vi "DecisionMaker.vi"(8 "Goal location":T3 {"North" format="%#_10f"; "East" format="%#_8f"}, 9 "Heading to test":dbl) -> (1 "Heading Goodness":T1)   [LabVIEW 2011]
doc: "VI to make decisions when the boat is headed upwind.\n\nCalculates the vector that goes to the goal from the boat's current location when first called.\nConstantly calculates the two optimal angles with respect to the wind and gives one of them as the optimal angle. On first call, this will be the one that is closer to the robot's current heading. It also calculates the distance from the boat to the original line calculated. If the distance gets larger than the allowed distance, it switches the angle outputted as optimal to the other angle that is good with respect to the wind."
uses:
  2 Typedefs/apparent wind direction.ctl
  2 Globals/2 TuningConstants.vi
  2 Globals/2 Global.vi
panel:
  in  "Irons direct vector":T2 {"Origin"."North" format="%#_10f"; "Origin"."East" format="%#_8f"}
  in  "Already Upwind?":bool
  # "0 < A < 1"
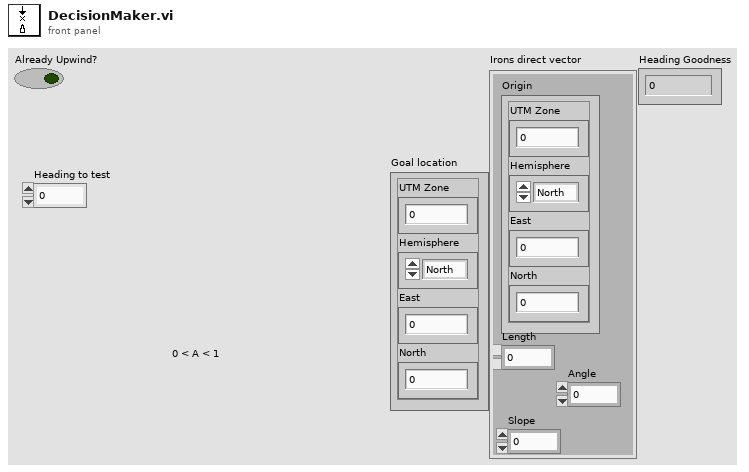
[diagram p1: front panel]
types:
  T1 = typedef "apparent wind direction.ctl" = dbl
  T2 = cluster{"Origin":cluster{"UTM Zone":dbl, "Hemisphere":enum16{"North", "South"}, "East":dbl, "North":dbl}, "Length":dbl, "Angle":dbl, "Slope":dbl}
  T3 = cluster{"UTM Zone":dbl, "Hemisphere":enum16{"North", "South"}, "East":dbl, "North":dbl}
  T4 = typedef "UTM Location.ctl" = cluster{"UTM Zone":dbl, "Hemisphere":enum16{"North", "South"}, "East":dbl, "North":dbl}
  T5 = cluster{"UTM Zone":bool, "Hemisphere":bool, "East":bool, "North":bool}
  T6 = typedef "heading.ctl" = dbl
  T7 = typedef "absolute wind direction.ctl" = dbl
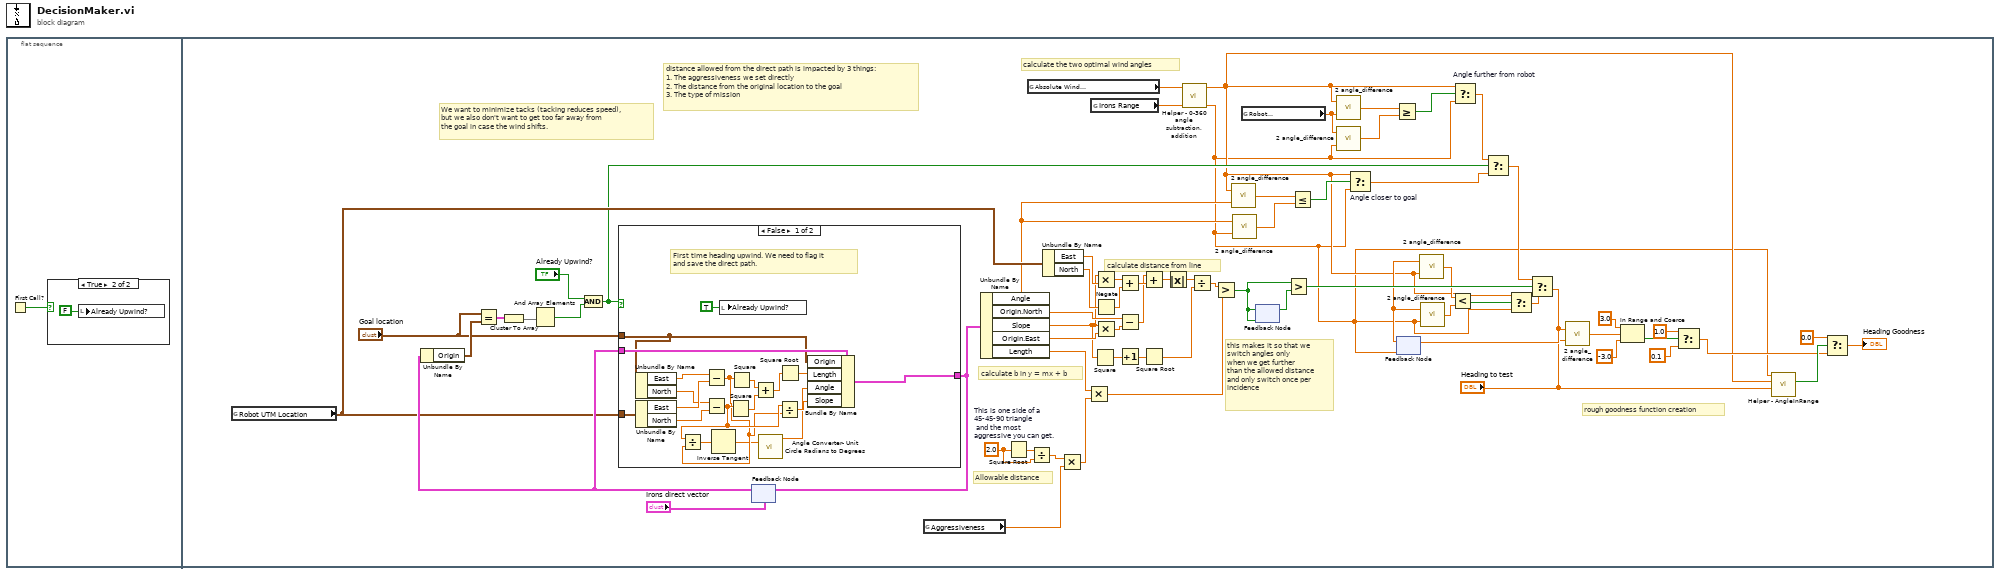
[diagram p0: block diagram]
diagram:
  n1 = flat-sequence {
    frame #0 {
      n2 = First Call?() -> (First Call?: T/F=w1:bool)
      n3 = case shown="True" w1 {
        frame False {
        }
        frame True {
          n4 = local write "Already Upwind?"(FALSE ("Already Upwind?")) -> ()
        }
      }
    }
    frame #1 {
      w47 = 2.0 ("x")
      # "Allowable distance"
      # "rough goodness function creation"
      # "this makes it so that we\nswitch angles only\nwhen we get further\nthan the allowed distance\nand only switch once per\nincidence"
      # "calculate distance from line"
      # "calculate the two optimal wind angles"
      # "calculate b in y = mx + b"
      # "distance allowed from the direct path is impacted by 3 things:\n1. The aggressiveness we set directly\n2. The distance from the original location to the goal\n3. The type of mission"
      # "We want to minimize tacks (tacking reduces speed),\nbut we also don't want to get too far away from\nthe goal in case the wind shifts."
      n5 = global read "2 Global.vi" "Robot UTM Location"() -> (w36:T4)
      n6 = feedback #1("Irons direct vector") -> (w45:T2)
      n7 = Unbundle By Name(w45) -> ("Origin"=w44:T3)
      n8 = Equal?(x="Goal location", y=w44) -> (x = y?=w43:T5)
      n9 = Cluster To Array(cluster=w43) -> (array=w42:bool[])
      n10 = And Array Elements(Boolean array=w42) -> (logical AND=w41:bool)
      n11 = And(x="Already Upwind?", y=w41) -> (x .and. y?=w13:bool)
      n12 = case shown="False" w13 {
        tunnel: w45 -> [w89 w91]
        tunnel: "Goal location" -> [w84 _]
        tunnel: w36 -> [w83 _]
        tunnel: [w77 w91] -> w55
        frame False {
          # "First time heading upwind. We need to flag it\nand save the direct path."
          n13 = Unbundle By Name(w84) -> ("East"=w82:dbl, "North"=w80:dbl)
          n14 = Unbundle By Name(w83) -> ("East"=w81:dbl, "North"=w79:dbl)
          n15 = Subtract(x=w82, y=w81) -> (x-y=w74:dbl)
          n16 = Subtract(x=w80, y=w79) -> (x-y=w75:dbl)
          n17 = Divide(x=w75, y=w74) -> (x/y=w78:dbl)
          n18 = Inverse Tangent(1:w78) -> (0:w73:dbl)
          n19 = local write "Already Upwind?"(TRUE ("Already Upwind?")) -> ()
          n20 = Square(x=w75) -> (x^2=w87:dbl)
          n21 = Square(x=w74) -> (x^2=w88:dbl)
          n22 = Add(x=w88, y=w87) -> (x+y=w85:dbl)
          n23 = call "Angle Converter- Unit Circle Radians to Degrees.vi"("Angle in \nUnit Circle\nRadians"=w73) -> ("Angle in \nHeading \nFormat"=w72:T6)  [unwired: 10 in]
          n24 = Divide(x=w75, y=w74) -> (x/y=w76:dbl)
          n25 = Square Root(x=w85) -> (sqrt(x)=w86:dbl)
          n26 = Bundle By Name(cluster=w89, "Origin"=w84, "Length"=w86, "Angle"=w72, "Slope"=w76) -> (w77:T2)
        }
        frame True {
        }
      }
      n27 = feedback-in #1(w55) -> ()
      n28 = global read "2 TuningConstants.vi" "Aggressiveness"() -> (w26:dbl)
      n29 = Unbundle By Name(w55) -> ("Angle"=w14:dbl, "Origin.North"=w70:dbl, "Slope"=w58:dbl, "Origin.East"=w69:dbl, "Length"=w50:dbl)
      n30 = Square Root(x=w47) -> (sqrt(x)=w48:dbl)
      n31 = global read "2 Global.vi" "Absolute Wind\nDirection (º)"() -> (w30:T7)
      n32 = Divide "This is one side of a 45-45-90 triangle\n and the most aggressive you can get."(x=w48, y=w47) -> (x/y=w29:dbl)
      n33 = Unbundle By Name(w36) -> ("East"=w67:dbl, "North"=w65:dbl)
      n34 = Multiply(x=w29, y=w26) -> (x*y=w28:dbl)
      n35 = Multiply(x=w50, y=w28) -> (x*y=w49:dbl)
      n36 = global read "2 TuningConstants.vi" "Irons Range"() -> (w31:dbl)
      n37 = Square(x=w58) -> (x^2=w57:dbl)
      n38 = Multiply(x=w58, y=w67) -> (x*y=w66:dbl)
      n39 = Negate(x=w65) -> (-x=w64:dbl)
      n40 = Multiply(x=w58, y=w69) -> (x*y=w68:dbl)
      n41 = Add(x=w66, y=w64) -> (x+y=w63:dbl)
      n42 = Subtract(x=w70, y=w68) -> (x-y=w62:dbl)
      n43 = Increment(x=w57) -> (x+1=w56:dbl)
      n44 = Add(x=w62, y=w63) -> (x+y=w61:dbl)
      n45 = Square Root(x=w56) -> (sqrt(x)=w59:dbl)
      n46 = Absolute Value(x=w61) -> (abs(x)=w60:dbl)
      n47 = call "Helper - 0-360 angle subtraction, addition.vi"("y"=w31, "x"=w30) -> ("x + y"=w4:dbl, "x - y"=w5:T1)  [unwired: 8 in]
      n48 = Divide(x=w60, y=w59) -> (x/y=w54:dbl)
      n49 = Greater?(x=w54, y=w49) -> (0:w34:bool)
      n50 = call "2 angle_difference.vi"("Angle 2"=w14, "Angle 1"=w5) -> ("Difference"=w16:dbl)
      n51 = call "2 angle_difference.vi"("Angle 2"=w4, "Angle 1"=w14) -> ("Difference"=w17:dbl)
      n52 = global read "2 Global.vi" "Robot\nHeading"() -> (w23:T6)
      n53 = feedback #2(w34) -> (w33:bool)
      n54 = feedback-in #2(w34) -> ()
      n55 = Greater?(x=w34, y=w33) -> (0:w32:bool)
      n56 = Less Or Equal?(x=w16, y=w17) -> (x <= y?=w15:bool)
      n57 = call "2 angle_difference.vi"("Angle 2"=w23, "Angle 1"=w5) -> ("Difference"=w24:dbl)
      n58 = call "2 angle_difference.vi"("Angle 2"=w4, "Angle 1"=w23) -> ("Difference"=w22:dbl)
      n59 = Select "Angle closer to goal"(t=w5, s=w15, f=w4) -> (s? t:f=w12:T1)
      n60 = Greater Or Equal?(x=w24, y=w22) -> (x >= y?=w25:bool)
      n61 = feedback #3(w4) -> (w9:T1)
      n62 = call "2 angle_difference.vi"("Angle 2"=w5, "Angle 1"=w9) -> ("Difference"=w7:dbl)
      n63 = call "2 angle_difference.vi"("Angle 2"=w4, "Angle 1"=w9) -> ("Difference"=w8:dbl)
      n64 = Less?(x=w7, y=w8) -> (x < y?=w6:bool)
      n65 = Select "Angle further from robot"(t=w5, s=w25, f=w4) -> (s? t:f=w11:T1)
      n66 = Select(t=w11, s=w13, f=w12) -> (s? t:f=w10:T1)
      n67 = Select(t=w5, s=w6, f=w4) -> (s? t:f=w3:T1)
      n68 = Select(t=w10, s=w32, f=w3) -> (s? t:f=w20:T1)
      n69 = feedback-in #3(w20) -> ()
      n70 = call "2 angle_difference.vi"("Angle 2"="Heading to test", "Angle 1"=w20) -> ("Difference"=w18:dbl)
      n71 = In Range and Coerce(upper limit=T1 3.0, x=w18, lower limit=T1 -3.0) -> (In Range?=w21:bool)  [unwired: 1 out]
      n72 = Select(t=1.0, s=w21, f=0.1) -> (s? t:f=w40:dbl)
      n73 = call "Helper - AngleInRange.vi"("Angle to check"="Heading to test", "Angle 2"=w5, "Angle 1"=w4) -> ("In range?"=w51:bool)  [unwired: 8 in]
      n74 = Select(t=0.0, s=w51, f=w40) -> (s? t:f=→"Heading Goodness":dbl)
    }
  }
